vi "GainMeasureAuto.vi"() -> ()   [LabVIEW 2020]
uses:
  <instrlib>/niScope/Controls/niScope vertical coupling.ctl
  <vilib>/Analysis/baseanly.llb/Mean (DBL).vi
  <instrlib>/niScope/Configure/Trigger/niScope Configure Trigger Immediate.vi
  <instrlib>/niScope/Acquire/Fetch/niScope Fetch.vi
  <userlib>/_OpenG.lib/time/time.llb/openg_time.lvlib
  <vilib>/Analysis/NI_AALBase.lvlib
panel:
  out "XY Graph":cluster{"V":dbl[], dbl[]}(graph)
  in  "V Step High":dbl=0.05
  in  "Aquire":bool
  in  "V Step low":dbl=0.2
  in  "Max V":dbl=4.6
  in  "Current V":dbl
  out "error out":errorcluster
  in  "Live":bool=TRUE
  out "Waveform Graph":dbl[](graph)
  in  "Channel":enum16{"Ch1", "Ch2", "Ch3"}(ring)
  in  "OK":bool
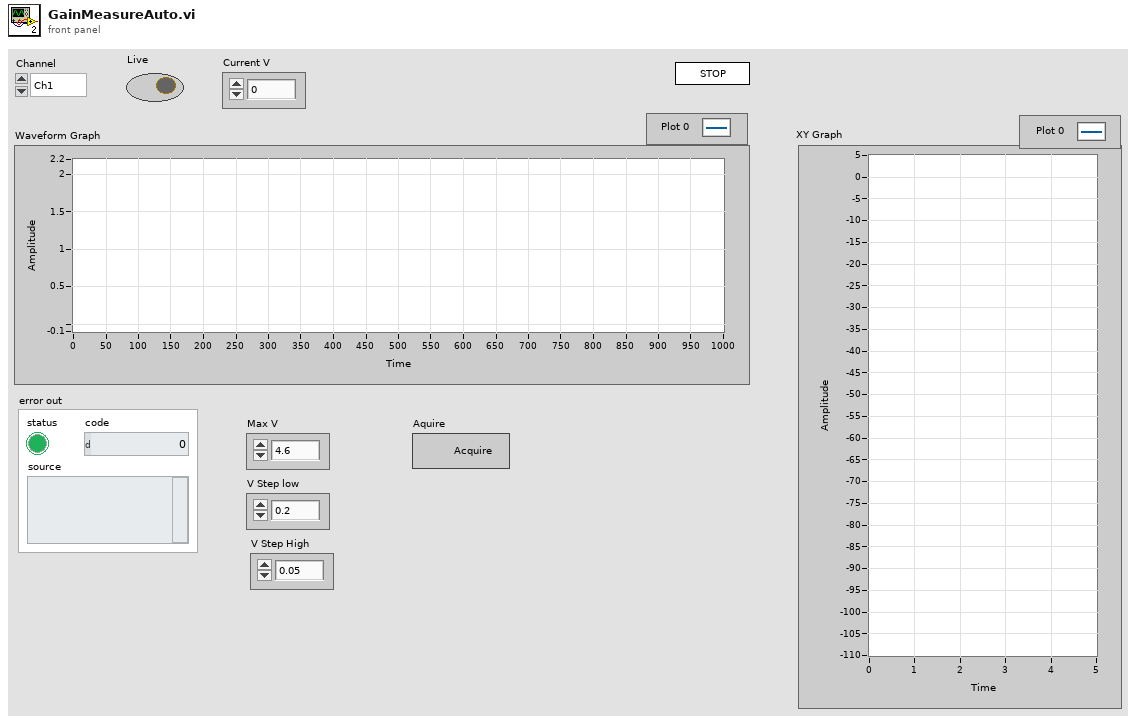
[diagram p1: front panel]
types:
  T1 = enum32{"Invalid", "Standard", "Closed", "Hidden", "Minimized", "Maximized"}
  T2 = enum32{"invalid app kind", "Development System", "Run Time System", "Student Edition", "Embedded LabVIEW", "Evaluation", "Custom"}
  T3 = enum16{"open", "open or create", "create or replace", "create", "open (read-only)"}
  T4 = cluster{"Core":cluster{"Current VI Reference":refnum<vi>, "Close Panel on Exit?":bool}, "Your Boolean data":bool, "Your string data":string, "Channel":enum16{"Ch1", "Ch2", "Ch3"}, "Digitizer":refnum<k15>, "Dig channels":string, "num points":i32, "LJ Handle":i32, "LJ pin":string, "V":dbl[], "wfm":dbl[][]}
  T5 = cluster{"Current VI Reference":refnum<vi>, "Close Panel on Exit?":bool}
  T6 = typedef "niScope vertical coupling.ctl" = i32
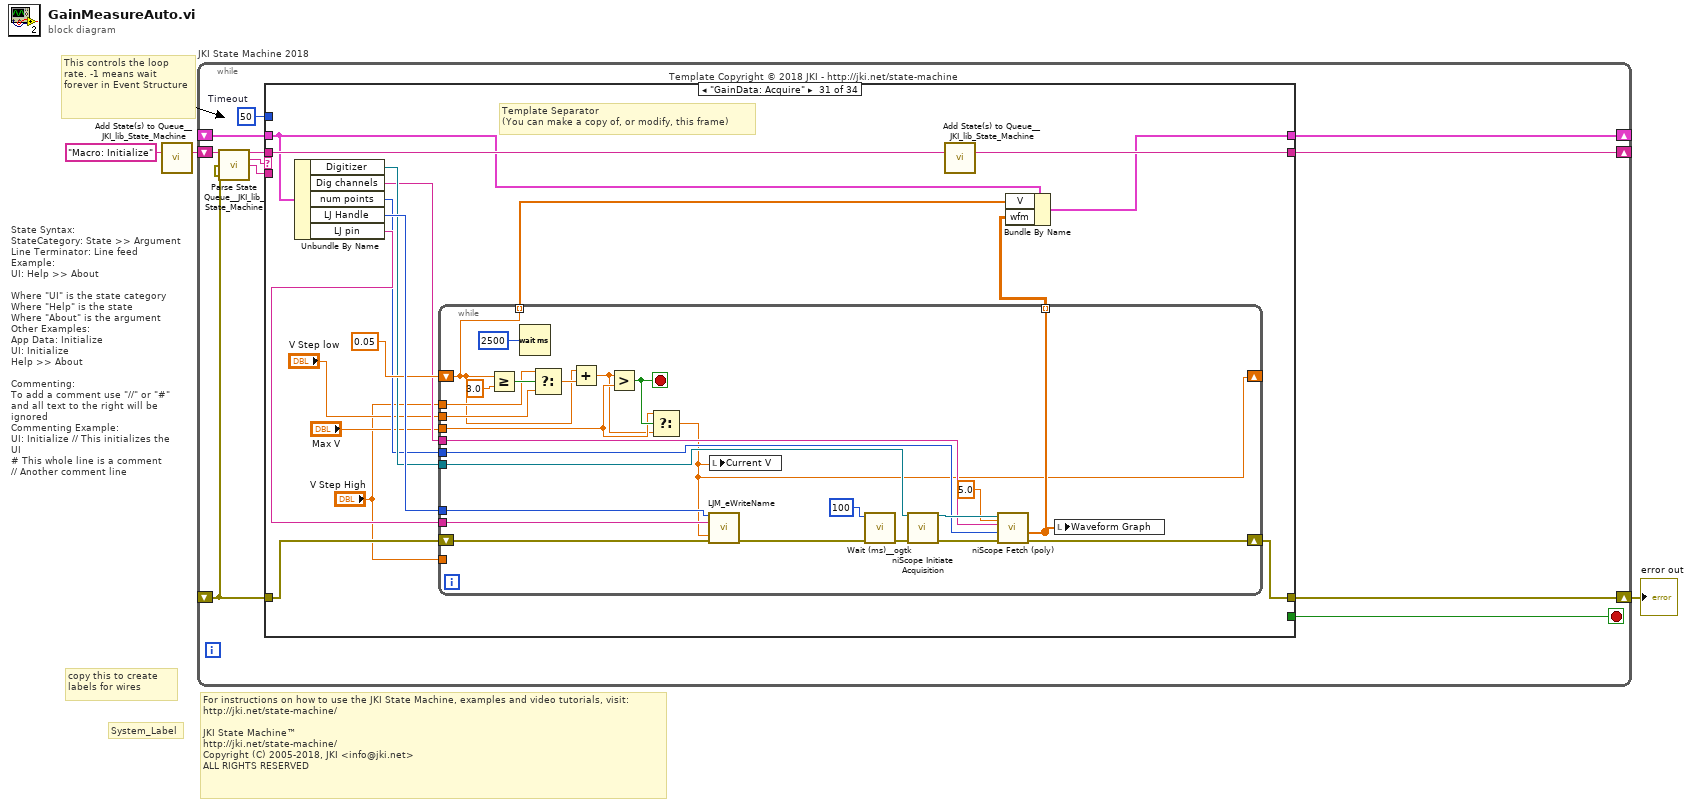
[diagram p0: block diagram]
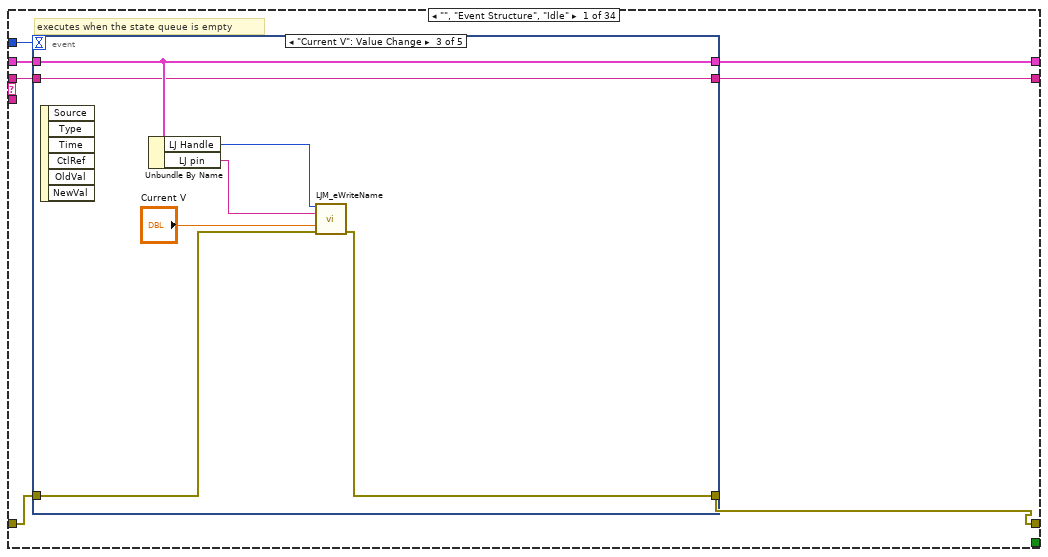
[diagram p2: hidden frame]
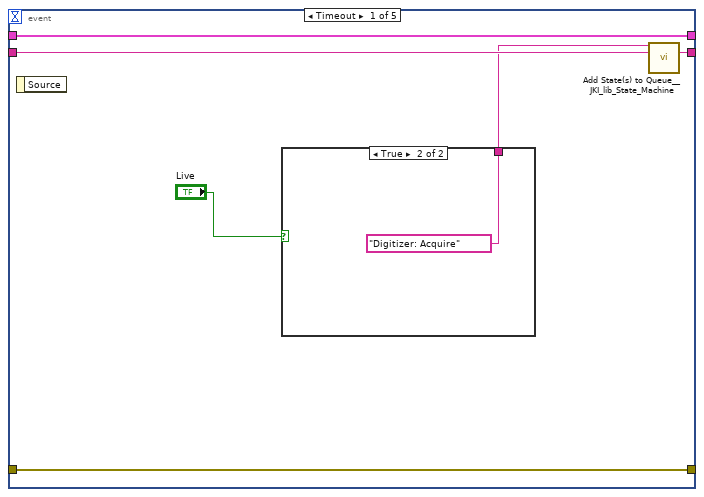
[diagram p3: hidden frame]
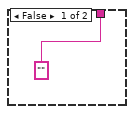
[diagram p4: hidden frame]
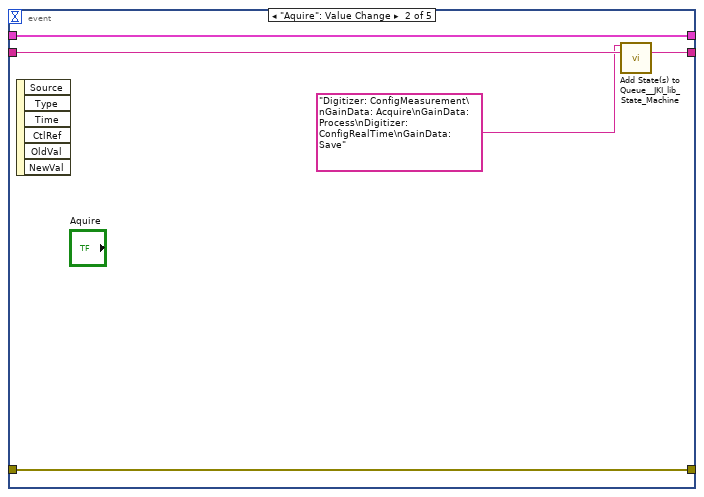
[diagram p5: hidden frame]
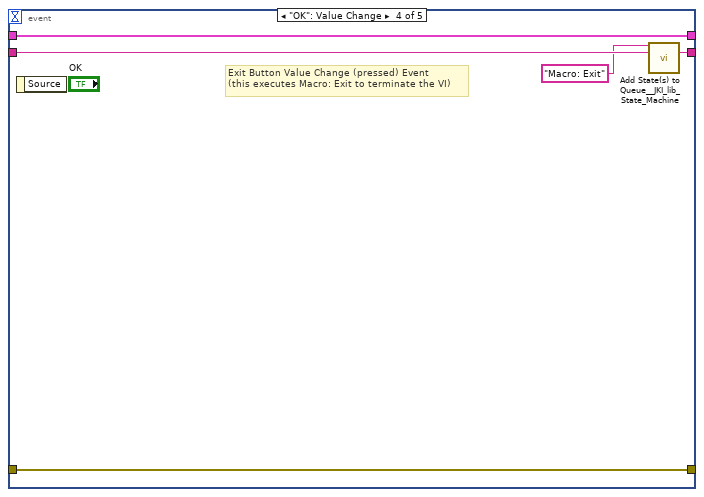
[diagram p6: hidden frame]
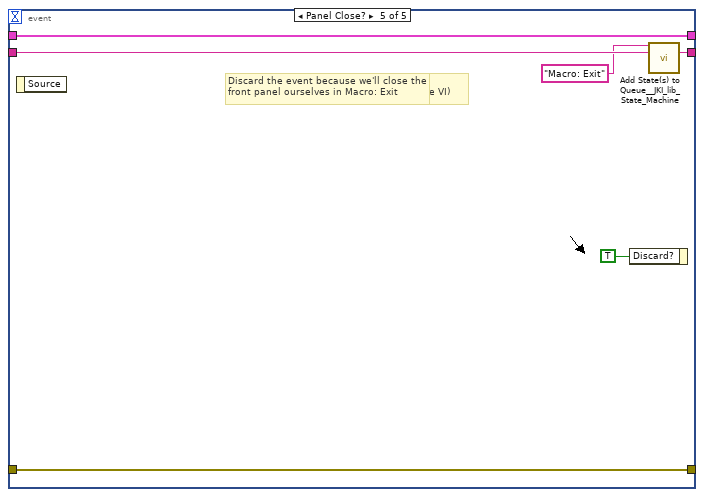
[diagram p7: hidden frame]
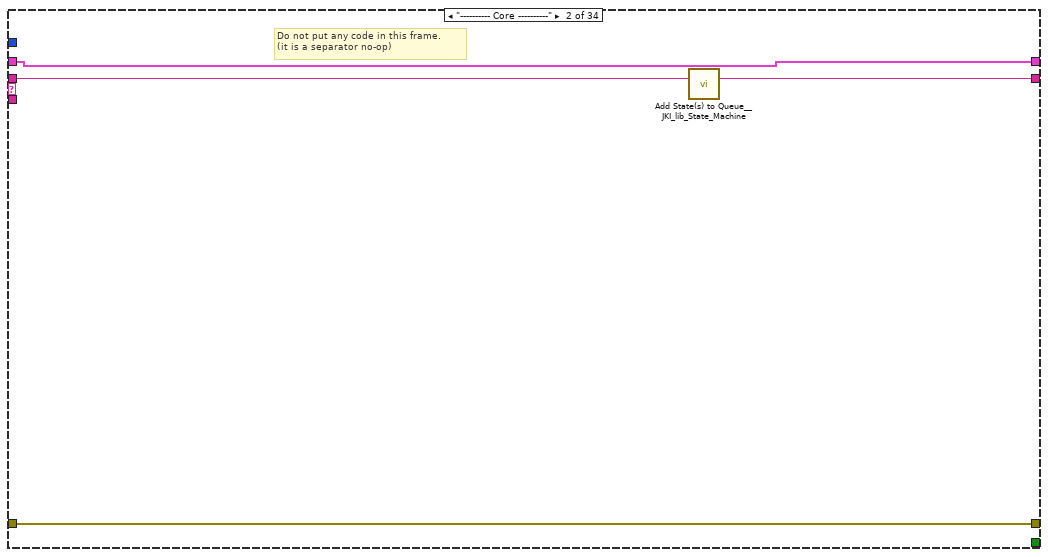
[diagram p8: hidden frame]
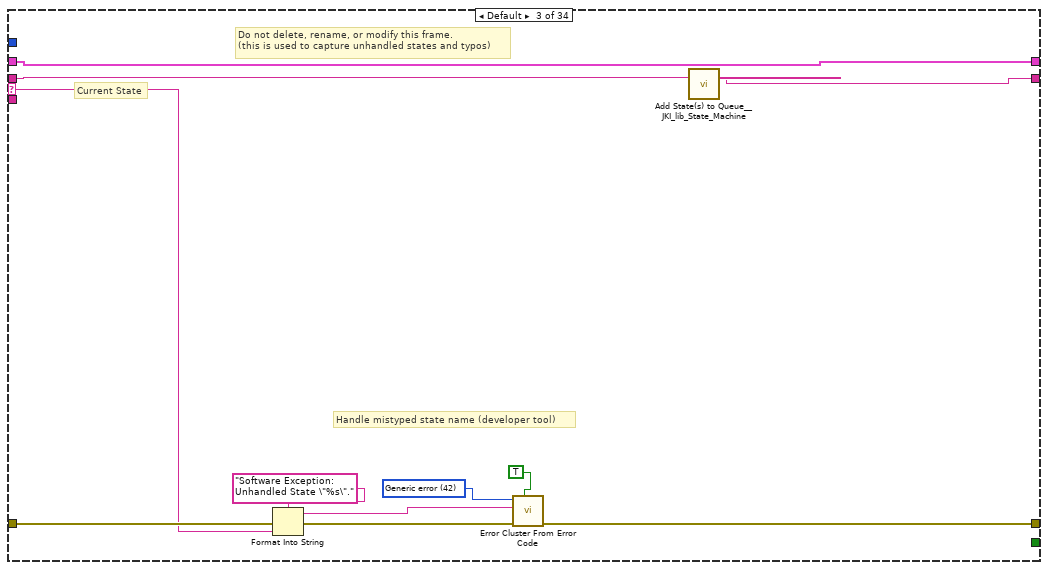
[diagram p9: hidden frame]
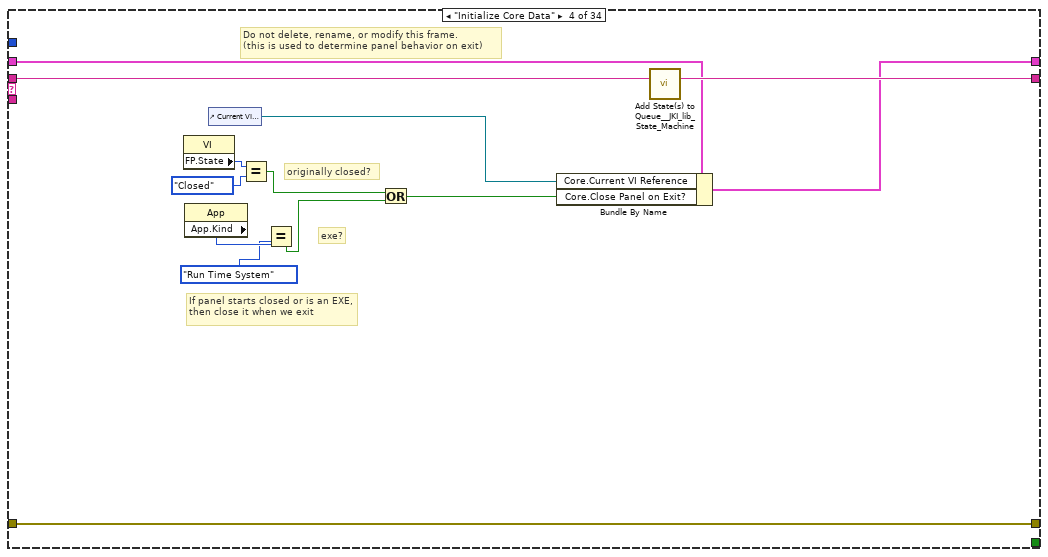
[diagram p10: hidden frame]
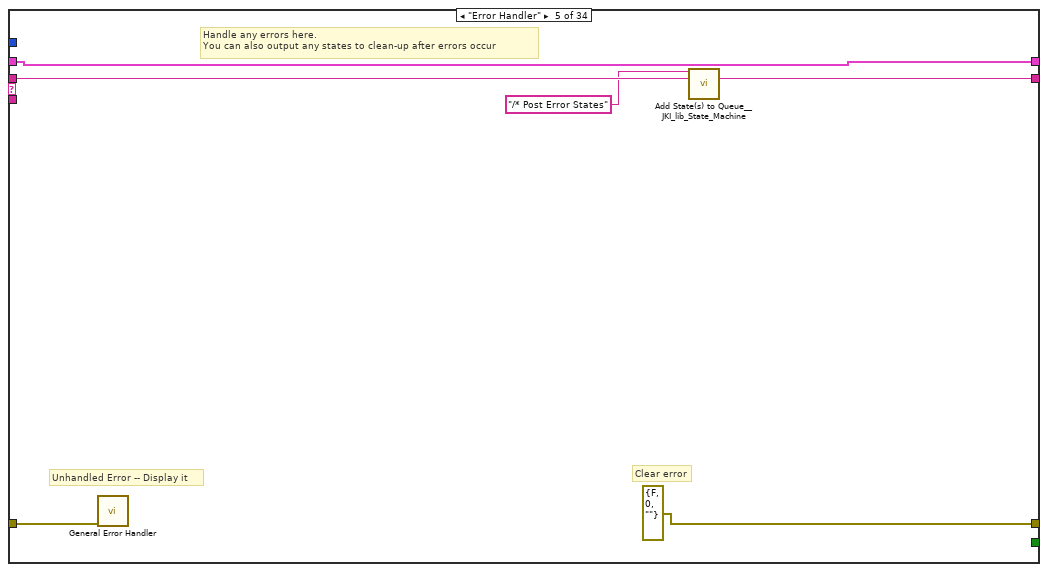
[diagram p11: hidden frame]
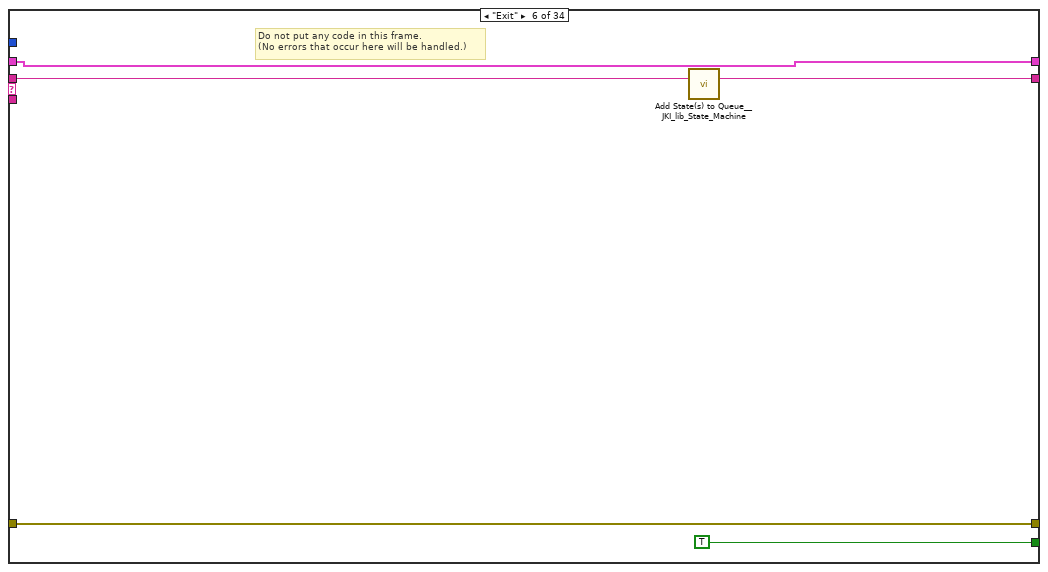
[diagram p12: hidden frame]
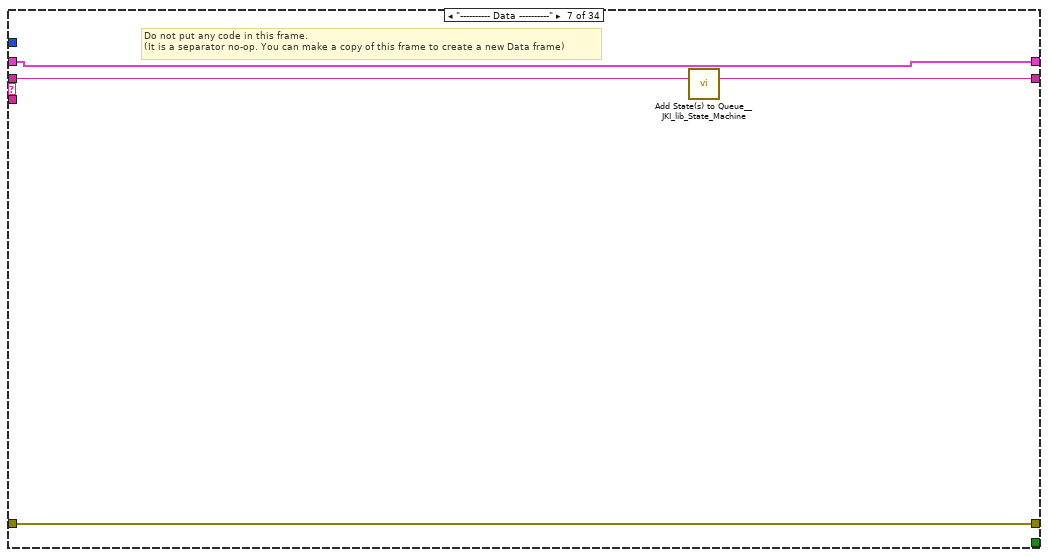
[diagram p13: hidden frame]
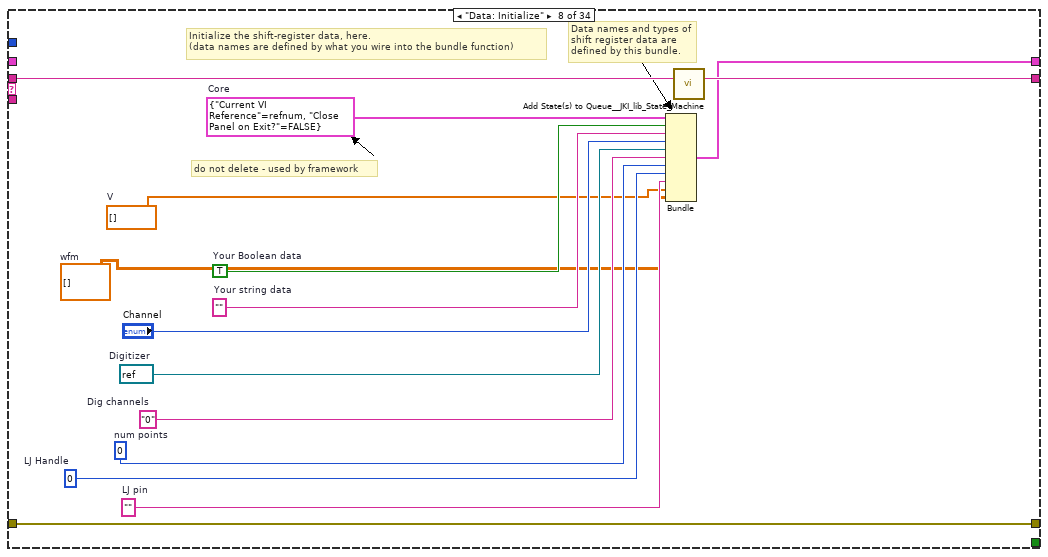
[diagram p14: hidden frame]
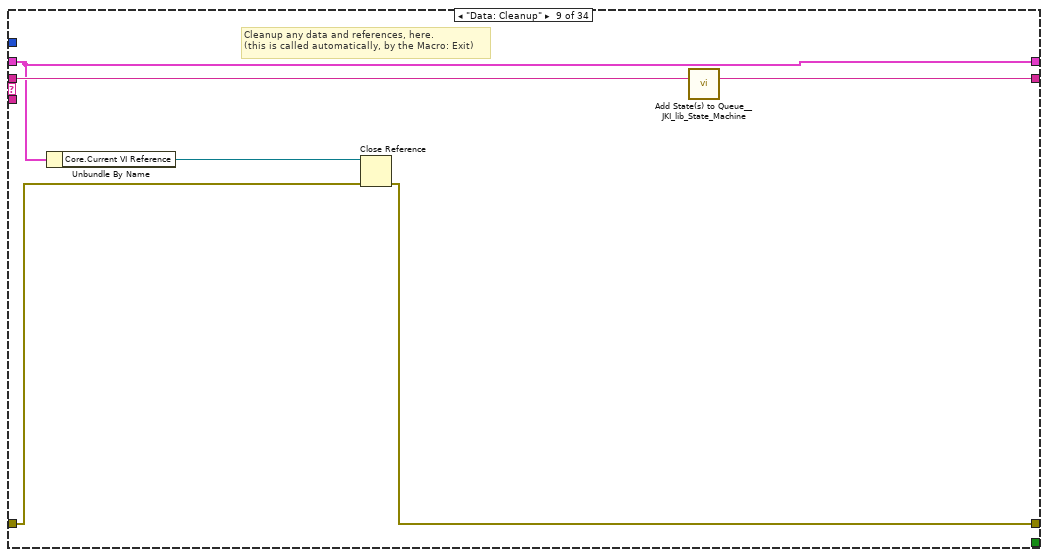
[diagram p15: hidden frame]
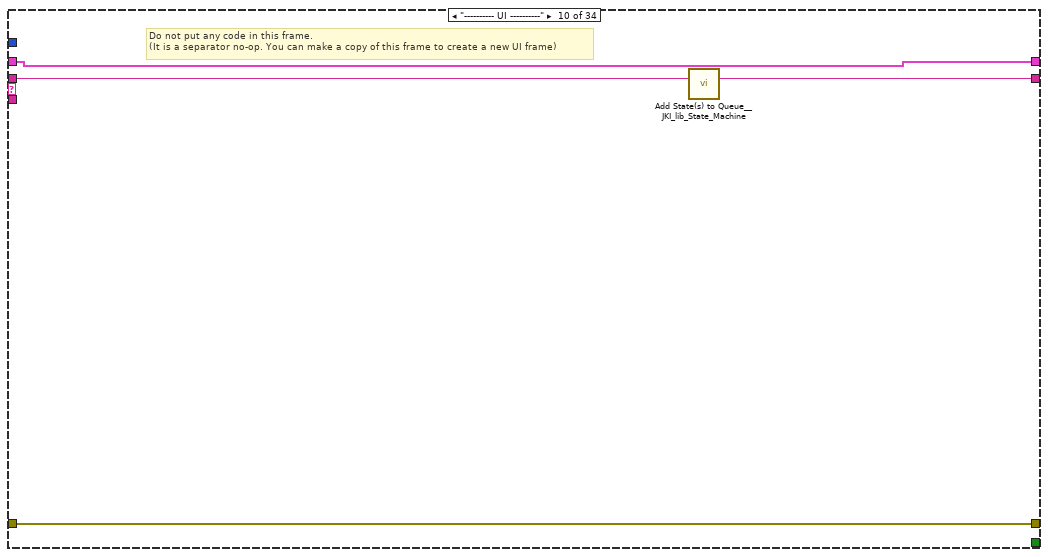
[diagram p16: hidden frame]
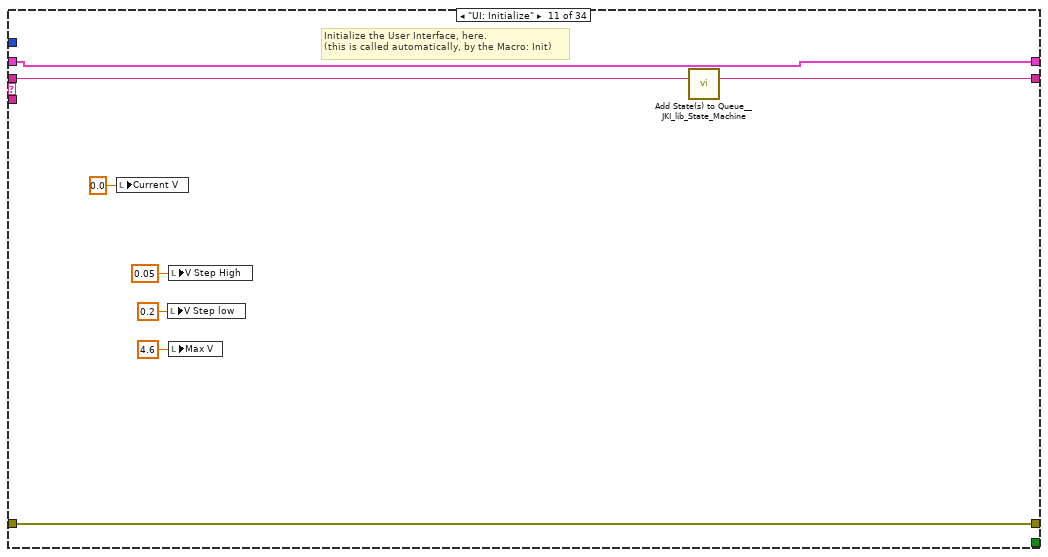
[diagram p17: hidden frame]
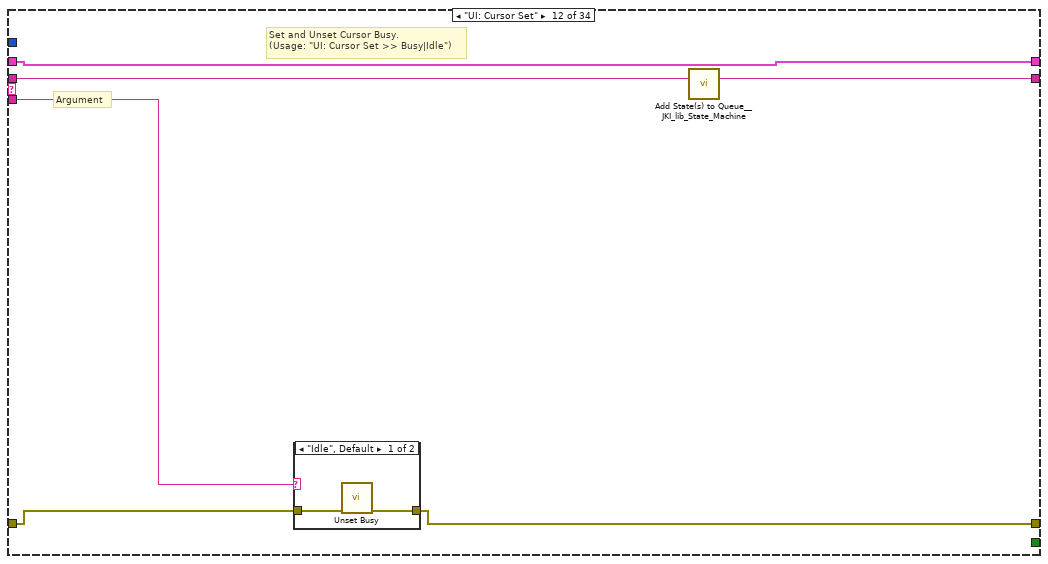
[diagram p18: hidden frame]
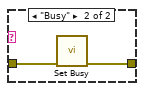
[diagram p19: hidden frame]
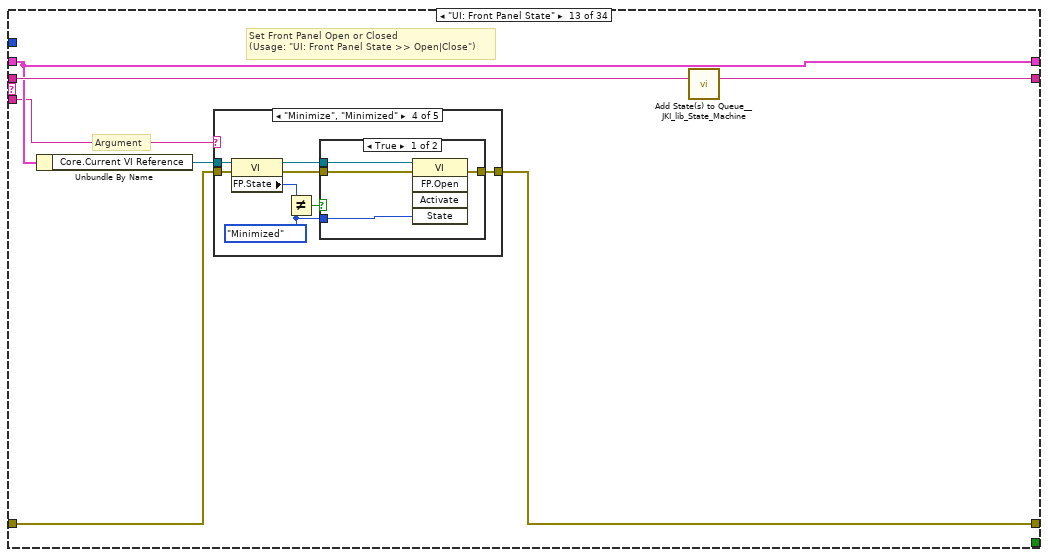
[diagram p20: hidden frame]
diagram:
  # "For instructions on how to use the JKI State Machine, examples and video tutorials, visit:\nhttp://jki.net/state-machine/\n\nJKI State Machine™\nhttp://jki.net/state-machine/\nCopyright (C) 2005-2018, JKI <info@jki.net>\nALL RIGHTS RESERVED"
  # "State Syntax:\nStateCategory: State >> Argument\nLine Terminator: Line feed\nExample:\nUI: Help >> About\n\nWhere \"UI\" is the state category\nWhere \"Help\" is the state\nWhere \"About\" is the argument\nOther Examples:\nApp Data: Initialize\nUI: Initialize\nHelp >> About\n\nCommenting:\nTo add a comment use \"//\" or \"#\" and all text to the right will be ignored\nCommenting Example:\nUI: Initialize // This initializes the UI\n# This whole line is a comment\n// Another comment line"
  # "copy this to create labels for wires"
  # "This controls the loop rate. -1 means wait forever in Event Structure"
  # "System_Label"
  n1 = call <vilib>:"Add State(s) to Queue__JKI_lib_State_Machine.vi"("State(s) in (\"\")"="Macro: Initialize") -> ("States Out"=w3:string)  [unwired: 14 in]
  n2 = while "JKI State Machine 2018" {
    shift-right: [w7] -> _
    shift-left: _ -> [w6]
    shift-right: [w10] -> w1
    shift-left: _ -> [w4]
    shift-right: [w9] -> _
    shift-left: w3 -> [w11]
    stop <- w8 stop-if-true
    w5 = 50  # Timeout
    # "Template Copyright © 2018 JKI - http://jki.net/state-machine"
    n3 = call <vilib>:"Parse State Queue__JKI_lib_State_Machine.vi"("State Queue"=w11, "Error In (no error)"=w4) -> ("Remaining States"=w13:string, "Current State"=w14:string, "Arguments"=w12:string)  [unwired: 11 in]
    n4 = case shown="\"GainData: Acquire\"" w14 {
      selector: w14 -> [_ _ w57 _ _ _ _ _ _ _ _ _ _ _ _ _ _ _ _ _ _ _ _ _ _ _ _ _ _ _ _ _ _ _]
      tunnel: w13 -> [w21 w56 w61 w80 w86 w91 w95 w110 w116 w120 w128 w134 w145 w214 w219 w229 w233 w242 w257 w283 w315 w332 w349 w353 w360 w368 w374 w378 w388 w417 w435 w464 w468 w472]
      tunnel: w12 -> [_ _ _ _ _ _ _ _ _ _ _ w129 w139 _ _ _ _ _ _ _ _ _ _ _ _ _ _ _ _ _ _ _ _ _]
      tunnel: w6 -> [w19 w53 w59 w73 w83 w89 w92 _ w111 w117 w126 w132 w141 w211 w216 w226 w230 w238 w253 w266 w298 w330 w347 w350 w355 w366 w372 w375 w385 w415 w422 w461 w465 w469]
      tunnel: [w18 w54 w63 w77 errorcluster {"status"=FALSE, "code"=0, "source"=""} ("error out") w88 w93 w107 w112 w118 w125 w130 w142 w212 w217 w227 w231 w240 w255 w268 w300 w327 w343 w351 w358 w362 w370 w376 w386 w398 w426 w462 w466 w470] -> w10
      tunnel: w4 -> [w17 w54 w62 w77 w82 w88 w93 w107 w113 w118 w125 w131 w143 w212 w217 w227 w231 w240 w254 w263 w292 w324 w342 w351 w357 w361 w369 w376 w386 w397 w427 w462 w466 w470]
      tunnel: [w20 w55 w60 w79 w85 w90 w94 w109 w115 w119 w127 w133 w144 w213 w218 w228 w232 w241 w256 w282 w314 w331 w348 w352 w359 w367 w373 w377 w387 w416 w434 w463 w467 w471] -> w9
      tunnel: [_ _ _ _ _ TRUE _ _ _ _ _ _ _ _ _ _ _ _ _ _ _ _ _ _ _ _ _ _ _ _ _ _ _ _] -> w8
      tunnel: [w16 w53 w59 w78 w83 w89 w92 w108 w111 w117 w126 w132 w141 w211 w216 w226 w230 w236 w253 w267 w299 w330 w347 w350 w356 w366 w372 w375 w385 w415 w423 w461 w465 w469] -> w7
      tunnel: w5 -> [w15 _ _ _ _ _ _ _ _ _ _ _ _ _ _ _ _ _ _ _ _ _ _ _ _ _ _ _ _ _ _ _ _ _]
      frame "", "Event Structure", "Idle" {
        # "executes when the state queue is empty"
        n5 = event shown="[2] \"Current V\": Value Change" {
          selector: _ -> [_ _ _ _ _]
          dyn-events: _ -> [_ _ _ _ _]
          timeout: w15 -> [_ _ _ _ _]
          tunnel: w21 -> [w27 w32 w35 w46 w52]
          tunnel: [w26 w33 w35 w45 w51] -> w20
          tunnel: w19 -> [w24 w34 w36 w43 w49]
          tunnel: [w25 w30 w37 w44 w50] -> w18
          tunnel: w17 -> [w25 w30 w38 w44 w50]
          tunnel: [w24 w34 w36 w43 w49] -> w16
          event Timeout {
            n6 = event-data() -> ()  [unwired: 1 in, 1 out]
            n7 = case shown="True" "Live" {
              tunnel: ["" ("State(s) in Front (\"\")") "Digitizer: Acquire" ("State(s) in Front (\"\")")] -> w22
              frame False {
              }
              frame True {
              }
            }
            n8 = call <vilib>:"Add State(s) to Queue__JKI_lib_State_Machine.vi"("State(s) in Front (\"\")"=w22, "State(s) in (\"\")"=w27) -> ("States Out"=w26:string)  [unwired: 13 in]
          }
          event "Aquire": Value Change {
            n9 = event-data() -> ()  [unwired: 1 in, 6 out]
            n10 = call <vilib>:"Add State(s) to Queue__JKI_lib_State_Machine.vi"("State(s) in Front (\"\")"="Digitizer: ConfigMeasurement\nGainData: Acquire\nGainData: Process\nDigitizer: ConfigRealTime\nGainData: Save" ("States Out"), "State(s) in (\"\")"=w32) -> ("States Out"=w33:string)  [unwired: 13 in]
          }
          event "Current V": Value Change {
            n11 = event-data() -> ()  [unwired: 1 in, 6 out]
            n12 = Unbundle By Name(w36) -> ("LJ Handle"=w41:i32, "LJ pin"=w40:string)
            n13 = call "LJM_eWriteName.vi"("Handle In"=w41, "Name"=w40, "Value"="Current V", "error in"=w38) -> ("error out"=w37:errorcluster)  [unwired: 10 in, 1 out]
          }
          event "OK": Value Change {
            # "Exit Button Value Change (pressed) Event\n(this executes Macro: Exit to terminate the VI)"
            n14 = event-data() -> ()  [unwired: 1 in, 1 out]
            n15 = call <vilib>:"Add State(s) to Queue__JKI_lib_State_Machine.vi"("State(s) in Front (\"\")"="Macro: Exit", "State(s) in (\"\")"=w46) -> ("States Out"=w45:string)  [unwired: 13 in]
          }
          event Panel Close? {
            # "Discard the event because we'll close the front panel ourselves in Macro: Exit"
            # "Close Panel button (pressed) Event\n(this executes Macro: Exit to terminate the VI)"
            n16 = event-data() -> ()  [unwired: 1 in, 1 out]
            n17 = event-data("Discard?"=TRUE) -> ()  [unwired: 1 in, 1 out]
            n18 = call <vilib>:"Add State(s) to Queue__JKI_lib_State_Machine.vi"("State(s) in Front (\"\")"="Macro: Exit", "State(s) in (\"\")"=w52) -> ("States Out"=w51:string)  [unwired: 13 in]
          }
        }
      }
      frame "---------- Core ----------" {
        # "Do not put any code in this frame.\n(it is a separator no-op)"
        n19 = call <vilib>:"Add State(s) to Queue__JKI_lib_State_Machine.vi"("State(s) in (\"\")"=w56) -> ("States Out"=w55:string)  [unwired: 14 in]
      }
      frame Default {
        w66 = 42 items=["No error", "Argument error", "Memory is full", "Out of zone", "End of file", "File already open", "Generic file I/O error", "File not found", "File permission error", "Disk is full", "Duplicate path", "Too many files open", "System feature not enabled", "Resource file not found", "Cannot add resource", "Resource not found", "Image not found", "Image memory error", "Pen does not exist", "Config type invalid", "Config token not found", "Config parse error", "Config memory error", "Bad external code format", "Bad external code offset", "External code not present", "Null window", "Destroy window error", "Null menu", "Print aborted", "Bad print record", "Print driver error", "Windows error during printing", "Memory error during printing", "Print dialog error", "Generic print error", "Invalid device refnum", "Device not found", "Device parameter error", "Device unit error", "Cannot open device", "Device call aborted", "Generic error", "Cancelled by user", "Object ID too low", "Object ID too high", "Object not in heap", "Unknown heap", "Unknown object (invalid DefProc)", "Unknown object (DefProc not in table)", "Message out of range", "Invalid (null) method", "Unknown message", "Manager call not supported", "Bad address", "Network operation in progress", "Network operation timed out", "Connection is busy", "Network attribute not supported", "Network error", "Address in use", "System out of memory", "Connection aborted", "Connection refused", "Not connected", "Already connected", "Connection closed", "Initialization error (interapplication manager)", "Bad occurrence", "Wait on unbound occurrence handler", "Occurrence queue overflow", "Datalog type conflict", "Unused", "Unrecognized type (interapplication manager)", "Memory corrupt", "Failed to make temporary DLL", "Old CIN version", "Drag socket not found", "Failed to load drop-object", "Failed to register OLE object", "Failed to release OLE object", "Format specifier type mismatch", "Unknown format specifier", "Too few format specifiers", "Too many format specifiers", "Scan failed", "Newer CIN version", "Error converting to variant", "Runtime menu error", "Password tampered", "Variant attribute not found", "Incompatible variant data type", "Event data is not available", "Event Store is not present", "Occurrence is not found", "Event Queue is not created", "Event info is not available", "Refnum passed is NULL", "Error retrieving Class GUID", "Error retrieving CoClass GUID", "Error retrieving TypeLib GUID.", "Bad built application magic bytes.", "Specific driver is different from the specific driver associated with the Logical Name.", "There is no session opened to the class driver.", "Max Error", "MAX - Error with config objects", "MAX - Error loading configuration", "MAX - Group not supported"]
        # "Current State"
        # "Do not delete, rename, or modify this frame.\n(this is used to capture unhandled states and typos)"
        # "Handle mistyped state name (developer tool)"
        n20 = Format Into String(format string="Software Exception: Unhandled State \"%s\"." ("message"), error in=w62, w57) -> (resulting string=w65:string, error out=w64:errorcluster)  [unwired: 1 in]
        n21 = call <vilib>:"Error Cluster From Error Code.vi"("show call chain? (False)"=TRUE, "error in (no error)"=w64, "error message (\"\")"=w65, "error code (0)"=w66) -> ("error out"=w63:errorcluster)  [unwired: 5 in]
        n22 = call <vilib>:"Add State(s) to Queue__JKI_lib_State_Machine.vi"("State(s) in (\"\")"=w61) -> ("States Out"=w60:string)  [unwired: 14 in]
      }
      frame "Initialize Core Data" {
        # "Do not delete, rename, or modify this frame.\n(this is used to determine panel behavior on exit)"
        # "originally closed?"
        # "exe?"
        # "If panel starts closed or is an EXE, then close it when we exit"
        n23 = property class="VI"() -> ("FP.State"=w70:T1)  [unwired: 2 in, 2 out]
        n24 = property class="App"() -> ("App.Kind"=w76:T2)  [unwired: 2 in, 2 out]
        n25 = control-ref of="Current VI Reference"() -> (w71:refnum<vi>)
        n26 = Equal?(x=w70, y=T1."Closed" ("Front Panel Window:State")) -> (x = y?=w68:bool)
        n27 = Equal?(x=w76, y=T2."Run Time System" ("Application:Kind")) -> (x = y?=w74:bool)
        n28 = Or(x=w68, y=w74) -> (x .or. y?=w72:bool)
        n29 = Bundle By Name(cluster=w73, "Core.Current VI Reference"=w71, "Core.Close Panel on Exit?"=w72) -> (w78:T4)
        n30 = call <vilib>:"Add State(s) to Queue__JKI_lib_State_Machine.vi"("State(s) in (\"\")"=w80) -> ("States Out"=w79:string)  [unwired: 14 in]
      }
      frame "Error Handler" {
        # "Unhandled Error -- Display it"
        # "Handle any errors here.\nYou can also output any states to clean-up after errors occur"
        # "Clear error"
        n31 = call <vilib>:"General Error Handler.vi"("error in (no error)"=w82) -> ()  [unwired: 10 in, 5 out]
        n32 = call <vilib>:"Add State(s) to Queue__JKI_lib_State_Machine.vi"("State(s) in Front (\"\")"="/* Post Error States", "State(s) in (\"\")"=w86) -> ("States Out"=w85:string)  [unwired: 13 in]
      }
      frame "Exit" {
        # "Do not put any code in this frame.\n(No errors that occur here will be handled.)"
        n33 = call <vilib>:"Add State(s) to Queue__JKI_lib_State_Machine.vi"("State(s) in (\"\")"=w91) -> ("States Out"=w90:string)  [unwired: 14 in]
      }
      frame "---------- Data ----------" {
        # "Do not put any code in this frame.\n(It is a separator no-op. You can make a copy of this frame to create a new Data frame)"
        n34 = call <vilib>:"Add State(s) to Queue__JKI_lib_State_Machine.vi"("State(s) in (\"\")"=w95) -> ("States Out"=w94:string)  [unwired: 14 in]
      }
      frame "Data: Initialize" {
        w96 = dbl[][] []  # wfm
        w97 = dbl[] []  # V
        w98 = ""  # LJ pin
        w99 = 0  # LJ Handle
        w100 = 0  # num points
        w101 = "0"  # Dig channels
        w102 = refnum<k15> refnum  # Digitizer
        w104 = T5 {"Current VI Reference"=refnum, "Close Panel on Exit?"=FALSE}  # Core
        w106 = TRUE  # Your Boolean data
        w105 = ""  # Your string data
        # "do not delete - used by framework"
        # "Data names and types of shift register data are defined by this bundle."
        # "Initialize the shift-register data, here.\n(data names are defined by what you wire into the bundle function)"
        n35 = Bundle("Core"=w104, "Your Boolean data"=w106, "Your string data"=w105, "Channel"="Channel", "Digitizer"=w102, "Dig channels"=w101, "num points"=w100, "LJ Handle"=w99, "LJ pin"=w98, "V"=w97, "wfm"=w96) -> (w108:T4)  [unwired: 1 in]
        n36 = call <vilib>:"Add State(s) to Queue__JKI_lib_State_Machine.vi"("State(s) in (\"\")"=w110) -> ("States Out"=w109:string)  [unwired: 14 in]
      }
      frame "Data: Cleanup" {
        # "Cleanup any data and references, here.\n(this is called automatically, by the Macro: Exit)"
        n37 = Unbundle By Name(w111) -> ("Core.Current VI Reference"=w114:refnum<vi>)
        n38 = Close Reference(reference=w114, error in (no error)=w113) -> (error out=w112:errorcluster)
        n39 = call <vilib>:"Add State(s) to Queue__JKI_lib_State_Machine.vi"("State(s) in (\"\")"=w116) -> ("States Out"=w115:string)  [unwired: 14 in]
      }
      frame "---------- UI ----------" {
        # "Do not put any code in this frame.\n(It is a separator no-op. You can make a copy of this frame to create a new UI frame)"
        n40 = call <vilib>:"Add State(s) to Queue__JKI_lib_State_Machine.vi"("State(s) in (\"\")"=w120) -> ("States Out"=w119:string)  [unwired: 14 in]
      }
      frame "UI: Initialize" {
        # "Initialize the User Interface, here.\n(this is called automatically, by the Macro: Init)"
        n41 = local write "Current V"(0.0 ("Current V")) -> ()
        n42 = local write "V Step low"(0.2 ("V Step low")) -> ()
        n43 = local write "V Step High"(0.05 ("V Step High")) -> ()
        n44 = local write "Max V"(4.6 ("Max V")) -> ()
        n45 = call <vilib>:"Add State(s) to Queue__JKI_lib_State_Machine.vi"("State(s) in (\"\")"=w128) -> ("States Out"=w127:string)  [unwired: 14 in]
      }
      frame "UI: Cursor Set" {
        # "Argument"
        # "Set and Unset Cursor Busy.\n(Usage: \"UI: Cursor Set >> Busy|Idle\")"
        n46 = case shown="\"Idle\", Default" w129 {
          tunnel: w131 -> [w136 w138]
          tunnel: [w135 w137] -> w130
          frame "Idle", Default {
            n47 = call <vilib>:"Unset Busy.vi"("error in (no error)"=w136) -> ("error out"=w135:errorcluster)  [unwired: 10 in]
          }
          frame "Busy" {
            n48 = call <vilib>:"Set Busy.vi"("error in (no error)"=w138) -> ("error out"=w137:errorcluster)  [unwired: 9 in, 1 out]
          }
        }
        n49 = call <vilib>:"Add State(s) to Queue__JKI_lib_State_Machine.vi"("State(s) in (\"\")"=w134) -> ("States Out"=w133:string)  [unwired: 14 in]
      }
      frame "UI: Front Panel State" {
        # "Argument"
        # "Set Front Panel Open or Closed\n(Usage: \"UI: Front Panel State >> Open|Close\")"
        n50 = Unbundle By Name(w141) -> ("Core.Current VI Reference"=w140:refnum<vi>)
        n51 = case shown="\"Minimize\", \"Minimized\"" w139 {
          tunnel: w143 -> [w151 w166 w177 w190 w203]
          tunnel: [w153 w167 w179 w192 w205] -> w142
          tunnel: w140 -> [w152 w164 w178 w191 w204]
          frame "Open", "Standard", Default {
            w146 = T1."Standard" ("State")
            n52 = property class="VI"(reference=w152, error in=w151) -> (reference out=w149:refnum<vi>, error out=w150:errorcluster, "FP.State"=w148:T1)
            n53 = Not Equal?(x=w148, y=w146) -> (x != y?=w147:bool)
            n54 = case shown="True" w147 {
              tunnel: [w157 w159] -> w153
              tunnel: w150 -> [w156 w159]
              tunnel: w149 -> [w155 _]
              tunnel: w146 -> [w154 _]
              frame True {
                n55 = invoke class="VI" method="FP.Open"(reference=w155, error in=w156, "Activate"=TRUE, "State"=w154) -> (error out=w157:errorcluster)  [unwired: 1 in, 4 out]
              }
              frame False {
              }
            }
          }
          frame "Close", "Closed" {
            n56 = property class="VI"(reference=w164, error in=w166) -> (reference out=w163:refnum<vi>, error out=w165:errorcluster, "FP.State"=w161:T1)
            n57 = Not Equal?(x=w161, y=T1."Closed" ("Front Panel Window:State")) -> (x != y?=w160:bool)
            n58 = case shown="True" w160 {
              tunnel: [w168 w171] -> w167
              tunnel: w165 -> [w168 w170]
              tunnel: w163 -> [_ w169]
              frame False {
              }
              frame True {
                n59 = invoke class="VI" method="FP.Close"(reference=w169, error in=w170) -> (error out=w171:errorcluster)  [unwired: 1 in, 2 out]
              }
            }
          }
          frame "Hidden", "Hide" {
            w172 = T1."Hidden" ("State")
            n60 = property class="VI"(reference=w178, error in=w177) -> (reference out=w175:refnum<vi>, error out=w176:errorcluster, "FP.State"=w174:T1)
            n61 = Not Equal?(x=w174, y=w172) -> (x != y?=w173:bool)
            n62 = case shown="True" w173 {
              tunnel: [w183 w184] -> w179
              tunnel: w176 -> [w182 w184]
              tunnel: w175 -> [w181 _]
              tunnel: w172 -> [w180 _]
              frame True {
                n63 = invoke class="VI" method="FP.Open"(reference=w181, error in=w182, "State"=w180) -> (error out=w183:errorcluster)  [unwired: 2 in, 4 out]
              }
              frame False {
              }
            }
          }
          frame "Minimize", "Minimized" {
            w185 = T1."Minimized" ("State")
            n64 = property class="VI"(reference=w191, error in=w190) -> (reference out=w188:refnum<vi>, error out=w189:errorcluster, "FP.State"=w187:T1)
            n65 = Not Equal?(x=w187, y=w185) -> (x != y?=w186:bool)
            n66 = case shown="True" w186 {
              tunnel: [w196 w197] -> w192
              tunnel: w189 -> [w195 w197]
              tunnel: w188 -> [w194 _]
              tunnel: w185 -> [w193 _]
              frame True {
                n67 = invoke class="VI" method="FP.Open"(reference=w194, error in=w195, "State"=w193) -> (error out=w196:errorcluster)  [unwired: 2 in, 4 out]
              }
              frame False {
              }
            }
          }
          frame "Maximize", "Maximized" {
            w198 = T1."Maximized" ("State")
            n68 = property class="VI"(reference=w204, error in=w203) -> (reference out=w201:refnum<vi>, error out=w202:errorcluster, "FP.State"=w200:T1)
            n69 = Not Equal?(x=w200, y=w198) -> (x != y?=w199:bool)
            n70 = case shown="True" w199 {
              tunnel: [w209 w210] -> w205
              tunnel: w202 -> [w208 w210]
              tunnel: w201 -> [w207 _]
              tunnel: w198 -> [w206 _]
              frame True {
                n71 = invoke class="VI" method="FP.Open"(reference=w207, error in=w208, "State"=w206) -> (error out=w209:errorcluster)  [unwired: 2 in, 4 out]
              }
              frame False {
              }
            }
          }
        }
        n72 = call <vilib>:"Add State(s) to Queue__JKI_lib_State_Machine.vi"("State(s) in (\"\")"=w145) -> ("States Out"=w144:string)  [unwired: 14 in]
      }
      frame "---------- Macro ----------" {
        # "Do not put any code in this frame.\n(It is a separator no-op. You can make a copy of this frame to create a new Macro frame)"
        n73 = call <vilib>:"Add State(s) to Queue__JKI_lib_State_Machine.vi"("State(s) in (\"\")"=w214) -> ("States Out"=w213:string)  [unwired: 14 in]
      }
      frame "Macro: Initialize" {
        # "Initialization Macro\n(This is called once, when the VI starts)"
        n74 = call <vilib>:"Add State(s) to Queue__JKI_lib_State_Machine.vi"("State(s) in Front (\"\")"="Data: Initialize\nInitialize Core Data\nUI: Initialize\nUI: Front Panel State >> Open\nDigitizer: Select\nDigitizer: Initilize\nDigitizer: ConfigRealTime\nLJ T7: Initialize\nLJ T7: setDefault", "State(s) in (\"\")"=w219) -> ("States Out"=w218:string)  [unwired: 13 in]
      }
      frame "Macro: Exit" {
        # "Exit Macro\n(This is called once, when the VI exits)"
        n75 = Unbundle By Name(w226) -> ("Core.Close Panel on Exit?"=w225:bool)
        n76 = Select(t="UI: Front Panel State >> Close", s=w225, f="") -> (s? t:f=w222:string)
        n77 = call <vilib>:"Add State(s) to Queue__JKI_lib_State_Machine.vi"("State(s) in (\"\")"=w222, "State(s) at Back (\"\")"="LJ T7: setDefault\nDigitizer: Close\nLJ T7: Close\nData: Cleanup\nExit") -> ("States Out"=w220:string)  [unwired: 13 in]
        n78 = call <vilib>:"Add State(s) to Queue__JKI_lib_State_Machine.vi"("State(s) in Front (\"\")"=w220, "State(s) in (\"\")"=w229) -> ("States Out"=w228:string)  [unwired: 13 in]
      }
      frame "---------- Digitizer ----------" {
        # "Template Separator\n(You can make a copy of, or modify, this frame)"
        n79 = call <vilib>:"Add State(s) to Queue__JKI_lib_State_Machine.vi"("State(s) in (\"\")"=w233) -> ("States Out"=w232:string)  [unwired: 14 in]
      }
      frame "Digitizer: Select" {
        # "Determin Digitizer\n(You can make a copy of, or modify, this frame)"
        n80 = Unbundle By Name(w238) -> ("Channel"=w239:enum16{"Ch1", "Ch2", "Ch3"})
        n81 = case shown="\"Ch3\"" w239 {
          tunnel: [w245 w248 w251] -> w237
          tunnel: ["0" ("Dig channels") "1" ("Dig channels") "0" ("Dig channels")] -> w235
          tunnel: ["TDAC13" ("LJ pin") "TDAC12" ("LJ pin") "DAC0" ("LJ pin")] -> w234
          frame "Ch1", Default {
            w245 = refnum<k15> "PXI1Slot3"  # Digitizer
          }
          frame "Ch2" {
            w248 = refnum<k15> "PXI1Slot3"  # Digitizer
          }
          frame "Ch3" {
            w251 = refnum<k15> "PXI1Slot4"  # Digitizer
          }
        }
        n82 = Bundle By Name(cluster=w238, "Digitizer"=w237, "Dig channels"=w235, "LJ pin"=w234) -> (w236:T4)
        n83 = call <vilib>:"Add State(s) to Queue__JKI_lib_State_Machine.vi"("State(s) in (\"\")"=w242) -> ("States Out"=w241:string)  [unwired: 14 in]
      }
      frame "Digitizer: Initilize" {
        # "Initialize Digitizer\n()"
        n84 = Unbundle By Name(w253) -> ("Digitizer"=w252:refnum<k15>)
        n85 = call <instrlib>:"niScope Initialize.vi"("resource name"=w252, "error in"=w254) -> ("error out"=w255:errorcluster)  [unwired: 12 in, 1 out]
        n86 = call <vilib>:"Add State(s) to Queue__JKI_lib_State_Machine.vi"("State(s) in (\"\")"=w257) -> ("States Out"=w256:string)  [unwired: 14 in]
      }
      frame "Digitizer: ConfigRealTime" {
        w276 = 100000.0 ("min sample rate")
        w278 = T6 1 items=["AC", "DC", "Ground"] ("vertical coupling")
        # "Template Separator\n(You can make a copy of, or modify, this frame)"
        n87 = Unbundle By Name(w266) -> ("Digitizer"=w264:refnum<k15>, "Dig channels"=w281:string)
        n88 = call <instrlib>:"niScope Acquisition Status.vi"("instrument handle"=w264, "error in"=w263) -> ("instrument handle out"=w261:refnum<k15>, "acquisition status"=w262:i32, "error out"=w259:errorcluster)  [unwired: 11 in]
        n89 = case shown="0, Default" w262 {
          tunnel: w261 -> [w287 w289]
          tunnel: [w286 w289] -> w260
          tunnel: w259 -> [w285 w288]
          tunnel: [w284 w288] -> w258
          frame 0, Default {
            n90 = call <instrlib>:"niScope Abort.vi"("instrument handle"=w287, "error in"=w285) -> ("instrument handle out"=w286:refnum<k15>, "error out"=w284:errorcluster)  [unwired: 12 in]
          }
          frame 1 {
          }
        }
        n91 = call <instrlib>:"niScope Configure Vertical.vi"("instrument handle"=w260, "vertical coupling"=w278, "channels"=w281, "vertical range"=2.0, "vertical offset"=1.0, "error in"=w258) -> ("instrument handle out"=w277:refnum<k15>, "error out"=w272:errorcluster)  [unwired: 8 in]
        n92 = Multiply(x=w276, y=0.01) -> (x*y=w265:dbl)
        n93 = Bundle By Name(cluster=w266, "num points"=w265) -> (w267:T4)
        n94 = call <instrlib>:"niScope Configure Horizontal Timing.vi"("instrument handle"=w277, "number of records"=1, "min sample rate"=w276, "error in"=w272, "min record length"=w265) -> ("instrument handle out"=w273:refnum<k15>, "error out"=w271:errorcluster)  [unwired: 9 in]
        n95 = call-poly <instrlib>:"niScope Configure Trigger (poly).vi"("instrument handle"=w273, "error in"=w271) -> ("instrument handle out"=w270:refnum<k15>, "error out"=w269:errorcluster)  [unwired: 12 in]
        n96 = call <instrlib>:"niScope Commit.vi"("instrument handle"=w270, "error in"=w269) -> ("error out"=w268:errorcluster)  [unwired: 12 in, 1 out]
        n97 = call <vilib>:"Add State(s) to Queue__JKI_lib_State_Machine.vi"("State(s) in (\"\")"=w283) -> ("States Out"=w282:string)  [unwired: 14 in]
      }
      frame "Digitizer: ConfigMeasurement" {
        w308 = 1000.0 ("min sample rate")
        w310 = T6 1 items=["AC", "DC", "Ground"] ("vertical coupling")
        # "Template Separator\n(You can make a copy of, or modify, this frame)"
        n98 = Unbundle By Name(w298) -> ("Digitizer"=w293:refnum<k15>, "Dig channels"=w313:string)
        n99 = call <instrlib>:"niScope Acquisition Status.vi"("instrument handle"=w293, "error in"=w292) -> ("instrument handle out"=w295:refnum<k15>, "acquisition status"=w296:i32, "error out"=w294:errorcluster)  [unwired: 11 in]
        n100 = case shown="0, Default" w296 {
          tunnel: w295 -> [w319 w321]
          tunnel: [w316 w321] -> w291
          tunnel: w294 -> [w318 w320]
          tunnel: [w317 w320] -> w290
          frame 0, Default {
            n101 = call <instrlib>:"niScope Abort.vi"("instrument handle"=w319, "error in"=w318) -> ("instrument handle out"=w316:refnum<k15>, "error out"=w317:errorcluster)  [unwired: 12 in]
          }
          frame 1 {
          }
        }
        n102 = call <instrlib>:"niScope Configure Vertical.vi"("instrument handle"=w291, "vertical coupling"=w310, "channels"=w313, "vertical range"=2.0, "vertical offset"=1.0, "error in"=w290) -> ("instrument handle out"=w309:refnum<k15>, "error out"=w304:errorcluster)  [unwired: 8 in]
        n103 = Multiply(x=w308, y=2.0) -> (x*y=w297:dbl)
        n104 = Bundle By Name(cluster=w298, "num points"=w297) -> (w299:T4)
        n105 = call <instrlib>:"niScope Configure Horizontal Timing.vi"("instrument handle"=w309, "number of records"=1, "min sample rate"=w308, "error in"=w304, "min record length"=w297) -> ("instrument handle out"=w305:refnum<k15>, "error out"=w303:errorcluster)  [unwired: 9 in]
        n106 = call-poly <instrlib>:"niScope Configure Trigger (poly).vi"("instrument handle"=w305, "error in"=w303) -> ("instrument handle out"=w302:refnum<k15>, "error out"=w301:errorcluster)  [unwired: 12 in]
        n107 = call <instrlib>:"niScope Commit.vi"("instrument handle"=w302, "error in"=w301) -> ("error out"=w300:errorcluster)  [unwired: 12 in, 1 out]
        n108 = call <vilib>:"Add State(s) to Queue__JKI_lib_State_Machine.vi"("State(s) in (\"\")"=w315) -> ("States Out"=w314:string)  [unwired: 14 in]
      }
      frame "Digitizer: Acquire" {
        # "Template Separator\n(You can make a copy of, or modify, this frame)"
        n109 = Unbundle By Name(w330) -> ("Digitizer"=w326:refnum<k15>, "Dig channels"=w329:string, "num points"=w328:i32)
        n110 = call <instrlib>:"niScope Acquisition Status.vi"("instrument handle"=w326, "error in"=w324) -> ("instrument handle out"=w323:refnum<k15>, "acquisition status"=w322:i32, "error out"=w325:errorcluster)  [unwired: 11 in]
        n111 = case shown="1" w322 {
          tunnel: w329 -> [_ w340]
          tunnel: w328 -> [_ w338]
          tunnel: [w333 w337] -> w327
          tunnel: w325 -> [w333 w335]
          tunnel: w323 -> [_ w334]
          frame 0, Default {
          }
          frame 1 {
            n112 = call <instrlib>:"niScope Initiate Acquisition.vi"("instrument handle"=w334, "error in"=w335) -> ("instrument handle out"=w341:refnum<k15>, "error out"=w339:errorcluster)  [unwired: 12 in]
            n113 = call-poly <instrlib>:"niScope Fetch (poly).vi"("error in"=w339, "numSamples"=w338, "channels"=w340, "instrument handle"=w341) -> ("error out"=w337:errorcluster, "wfm"=→"Waveform Graph":dbl[])  [unwired: 4 in, 2 out]
          }
        }
        n114 = call <vilib>:"Add State(s) to Queue__JKI_lib_State_Machine.vi"("State(s) in (\"\")"=w332) -> ("States Out"=w331:string)  [unwired: 14 in]
      }
      frame "Digitizer: Close" {
        # "Template Separator\n(You can make a copy of, or modify, this frame)"
        n115 = Unbundle By Name(w347) -> ("Digitizer"=w346:refnum<k15>)
        n116 = call <instrlib>:"niScope Abort.vi"("instrument handle"=w346, "error in"=w342) -> ("instrument handle out"=w345:refnum<k15>, "error out"=w344:errorcluster)  [unwired: 12 in]
        n117 = call <instrlib>:"niScope Close.vi"("instrument handle"=w345, "error in"=w344) -> ("error out"=w343:errorcluster)  [unwired: 13 in]
        n118 = call <vilib>:"Add State(s) to Queue__JKI_lib_State_Machine.vi"("State(s) in (\"\")"=w349) -> ("States Out"=w348:string)  [unwired: 14 in]
      }
      frame "---------- LJ T7 ----------" {
        # "Template Separator\n(You can make a copy of, or modify, this frame)"
        n119 = call <vilib>:"Add State(s) to Queue__JKI_lib_State_Machine.vi"("State(s) in (\"\")"=w353) -> ("States Out"=w352:string)  [unwired: 14 in]
      }
      frame "LJ T7: Initialize" {
        # "Template Separator\n(You can make a copy of, or modify, this frame)"
        n120 = call "LJ_Open.vi"("error in"=w357) -> ("error out"=w358:errorcluster, "Handle Out"=w354:i32)  [unwired: 8 in, 1 out]
        n121 = Bundle By Name(cluster=w355, "LJ Handle"=w354) -> (w356:T4)
        n122 = call <vilib>:"Add State(s) to Queue__JKI_lib_State_Machine.vi"("State(s) in (\"\")"=w360) -> ("States Out"=w359:string)  [unwired: 14 in]
      }
      frame "LJ T7: setDefault" {
        # "Template Separator\n(You can make a copy of, or modify, this frame)"
        n123 = Unbundle By Name(w366) -> ("LJ Handle"=w365:i32, "LJ pin"=w364:string)
        n124 = call "LJM_eWriteName.vi"("Handle In"=w365, "Name"=w364, "Value"=0.0, "error in"=w361) -> ("error out"=w362:errorcluster)  [unwired: 10 in, 1 out]
        n125 = call <vilib>:"Add State(s) to Queue__JKI_lib_State_Machine.vi"("State(s) in (\"\")"=w368) -> ("States Out"=w367:string)  [unwired: 14 in]
      }
      frame "LJ T7: Close" {
        # "Template Separator\n(You can make a copy of, or modify, this frame)"
        n126 = Unbundle By Name(w372) -> ("LJ Handle"=w371:i32)
        n127 = call "LJM_Close.vi"("error in"=w369, "Handle"=w371) -> ("error out"=w370:errorcluster)  [unwired: 9 in]
        n128 = call <vilib>:"Add State(s) to Queue__JKI_lib_State_Machine.vi"("State(s) in (\"\")"=w374) -> ("States Out"=w373:string)  [unwired: 14 in]
      }
      frame "---------- GainData ----------" {
        # "Template Separator\n(You can make a copy of, or modify, this frame)"
        n129 = call <vilib>:"Add State(s) to Queue__JKI_lib_State_Machine.vi"("State(s) in (\"\")"=w378) -> ("States Out"=w377:string)  [unwired: 14 in]
      }
      frame "GainData: Process" {
        # "Template Separator\n(You can make a copy of, or modify, this frame)"
        n130 = Unbundle By Name(w385) -> ("V"=w383:dbl[], "wfm"=w384:dbl[][])
        n131 = for {
          tunnel: w384 -> [w393] mode=indexing
          tunnel: [w392] -> w380 mode=indexing
          # "Avergae"
          n132 = call-poly <vilib>:"Mean.vi"("X"=w393) -> ("mean"=w392:dbl)  [unwired: 1 out]
        }
        n133 = Index Array(array=w380) -> (element=w381:dbl)  [unwired: 1 in]
        n134 = for {
          tunnel: w381 -> [w390]
          tunnel: w380 -> [w391] mode=indexing
          tunnel: [w389] -> w379 mode=indexing
          # "Nomalize"
          n135 = Divide(x=w391, y=w390) -> (x/y=w389:dbl)
        }
        n136 = Bundle("V"=w383, w379) -> (→"XY Graph":cluster{"V":dbl[], dbl[]})  [unwired: 1 in]
        n137 = call <vilib>:"Add State(s) to Queue__JKI_lib_State_Machine.vi"("State(s) in (\"\")"=w388) -> ("States Out"=w387:string)  [unwired: 14 in]
      }
      frame "GainData: Save" {
        # "Template Separator\n(You can make a copy of, or modify, this frame)"
        n138 = Current VI's Path() -> (path=w395:path)
        n139 = call "File Dialog"("start path"=w395, "default name"="GainSweep") -> ("selected path"=w396:path)  [unwired: 10 in, 3 out]
        n140 = Unbundle By Name(w415) -> ("V"=w402:dbl[], "wfm"=w407:dbl[][])
        n141 = TDMS Open(8:w397, 10:T3."create or replace" ("operation (0:open)"), 11:w396) -> (0:w410:errorcluster, 3:w413:refnum<k34>)  [unwired: 4 in]
        n142 = Array Size(array=w407) -> (size(s)=w411:i32[])
        n143 = TDMS Set Properties(5:w411, 7:string[] ["Num of points", "Data Length"] ("property names"), 8:w410, 11:w413) -> (0:w408:errorcluster, 3:w409:refnum<k34>)  [unwired: 2 in, 2 out]
        n144 = for {
          tunnel: w407 -> [w418] mode=indexing
          tunnel: [w418] -> w406 mode=concatenating
          # "Reshape"
        }
        n145 = TDMS Write(0:w409, 7:string[] ["Voltage"] ("channel name(s) in (Untitled)"), 9:w406, 11:w408) -> (4:w404:refnum<k34>, 15:w403:errorcluster)  [unwired: 2 in, 2 out]
        n146 = TDMS Write(0:w404, 7:string[] ["V"] ("channel name(s) in (Untitled)"), 9:w402, 11:w403) -> (4:w400:refnum<k34>, 15:w399:errorcluster)  [unwired: 2 in, 2 out]
        n147 = call <vilib>:"Add State(s) to Queue__JKI_lib_State_Machine.vi"("State(s) in (\"\")"=w417) -> ("States Out"=w416:string)  [unwired: 14 in]
        n148 = TDMS Close(8:w399, 11:w400) -> (0:w398:errorcluster)  [unwired: 1 out]
      }
      frame "GainData: Acquire" {
        # "Template Separator\n(You can make a copy of, or modify, this frame)"
        n149 = Unbundle By Name(w422) -> ("Digitizer"=w430:refnum<k15>, "Dig channels"=w429:string, "num points"=w428:i32, "LJ Handle"=w433:i32, "LJ pin"=w432:string)
        n150 = while {
          tunnel: w433 -> [w460]
          tunnel: w432 -> [w459]
          shift-right: [w436] -> _
          shift-left: 0.05 -> [w441]
          tunnel: w430 -> [w456]
          tunnel: w429 -> [w454]
          tunnel: w428 -> [w453]
          shift-right: [w448] -> w426
          shift-left: w427 -> [w458]
          tunnel: "V Step High" -> [w444]
          tunnel: "V Step low" -> [w443]
          tunnel: "Max V" -> [w438]
          tunnel: [w441] -> w421 mode=indexing
          tunnel: [w440] -> w420 mode=indexing
          tunnel: "V Step High" -> [_]
          stop <- w439 stop-if-true
          n151 = Greater Or Equal?(x=w441, y=3.0) -> (x >= y?=w445:bool)
          n152 = Wait (ms)(milliseconds to wait=u32 2500) -> ()  [unwired: 1 out]
          n153 = Select(t=w444, s=w445, f=w443) -> (s? t:f=w442:dbl)
          n154 = Add(x=w441, y=w442) -> (x+y=w437:dbl)
          n155 = Greater?(x=w437, y=w438) -> (0:w439:bool)
          n156 = Select(t=w438, s=w439, f=w437) -> (s? t:f=w436:dbl)
          n157 = call "LJM_eWriteName.vi"("Handle In"=w460, "Name"=w459, "Value"=w436, "error in"=w458) -> ("error out"=w457:errorcluster)  [unwired: 10 in, 1 out]
          n158 = local write "Current V"(w436) -> ()
          n159 = call <userlib>:"Wait (ms)__ogtk.vi"("error in (no error)"=w457, "milliseconds to wait"=u32 100) -> ("error out"=w451:errorcluster)  [unwired: 8 in, 1 out]
          n160 = call <instrlib>:"niScope Initiate Acquisition.vi"("instrument handle"=w456, "error in"=w451) -> ("instrument handle out"=w455:refnum<k15>, "error out"=w452:errorcluster)  [unwired: 12 in]
          n161 = call-poly <instrlib>:"niScope Fetch (poly).vi"("timeout"=5.0, "error in"=w452, "numSamples"=w453, "channels"=w454, "instrument handle"=w455) -> ("error out"=w448:errorcluster, "wfm"=w440:dbl[])  [unwired: 3 in, 2 out]
          n162 = local write "Waveform Graph"(w440) -> ()
        }
        n163 = call <vilib>:"Add State(s) to Queue__JKI_lib_State_Machine.vi"("State(s) in (\"\")"=w435) -> ("States Out"=w434:string)  [unwired: 14 in]
        n164 = Bundle By Name(cluster=w422, "V"=w421, "wfm"=w420) -> (w423:T4)
      }
      frame "---------- New Category ----------" {
        # "Template Separator\n(You can make a copy of, or modify, this frame)"
        n165 = call <vilib>:"Add State(s) to Queue__JKI_lib_State_Machine.vi"("State(s) in (\"\")"=w464) -> ("States Out"=w463:string)  [unwired: 14 in]
      }
      frame "New Category: 1" {
        # "Your code here.\n(You can make a copy of, or modify, this frame)"
        n166 = call <vilib>:"Add State(s) to Queue__JKI_lib_State_Machine.vi"("State(s) in (\"\")"=w468) -> ("States Out"=w467:string)  [unwired: 14 in]
      }
      frame "New Category: 2" {
        # "Your code here.\n(You can make a copy of, or modify, this frame)"
        n167 = call <vilib>:"Add State(s) to Queue__JKI_lib_State_Machine.vi"("State(s) in (\"\")"=w472) -> ("States Out"=w471:string)  [unwired: 14 in]
      }
    }
  }
  "error out" <- w1
